vi "CH_LM DataString2StreamingCluster.vi"(3 "error in (no error)":errorcluster, 4 "Data Strings":string[](array[string]), 5 "Meter Index":i32) -> (0 "error out":errorcluster, 1 "Data Array":T1[](array[typedef]) {"Flags" format="%.0b"; "Unit ID" format="%.0b"; "Quad Distance"."Y" format="%#.1f"; "Quad Distance"."X" format="%#.1f"; "Value" format="%#.7e"}, 2 "Meter Index out":i32)   [LabVIEW 2017, in "CH_LM.lvlib"]
doc: "This VI converts the received data record strings to an array of Streaming Data Cluster."
uses:
  CH_LM.lvlib
  CH_LM/CH_LM Streaming Data.ctl
  CH_LM/CH_LM Data Token.ctl
panel:
  in  "Steaming Data Cluster":T1 {"Flags" format="%.0b"; "Unit ID" format="%.0b"; "Quad Distance"."Y" format="%#.1f"; "Quad Distance"."X" format="%#.1f"; "Value" format="%#.7e"}
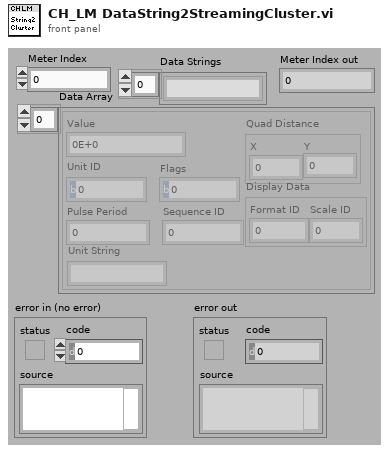
[diagram p1: front panel]
types:
  T1 = typedef "CH_LM.lvlib/CH_LM Streaming Data.ctl" = cluster{"Value":sgl, "Quad Distance":cluster{"X":sgl, "Y":sgl}, "Display Data":cluster{"Format ID":u8, "Scale ID":u8}, "Unit ID":u8, "Flags":u32, "Pulse Period":u32, "Sequence ID":u32, "Unit String":string}
  T2 = typedef "CH_LM.lvlib/CH_LM Data Token.ctl" = enum16{"Raw data", "Quad distance", "Formated data", "Unit", "Pulse period", "Flags", "Sequence ID"}
  T3 = typedef "CH_LM.lvlib/CH_LM Meter Info.ctl" = cluster{"Meter Index":i32, "Serial Number":string, "Queue Cluster":T4, "Data Header":bool, "Data Tokens":T2[]}
  T4 = typedef "CH_LM.lvlib/CH_LM Queue Cluster.ctl" = cluster{"Streaming Queue":refnum<queue>, "Asynch Notifier":refnum<notifier>}
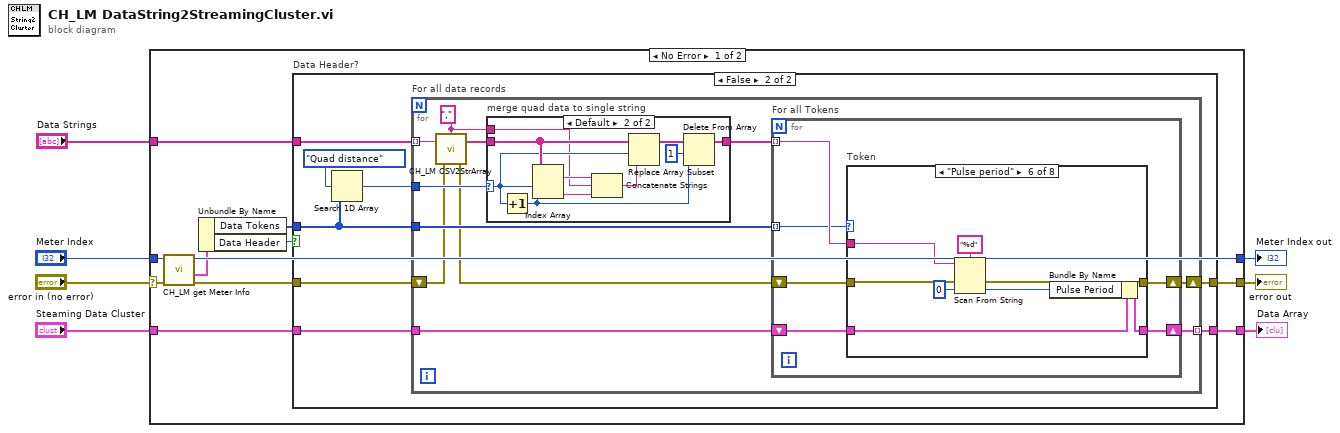
[diagram p0: block diagram]
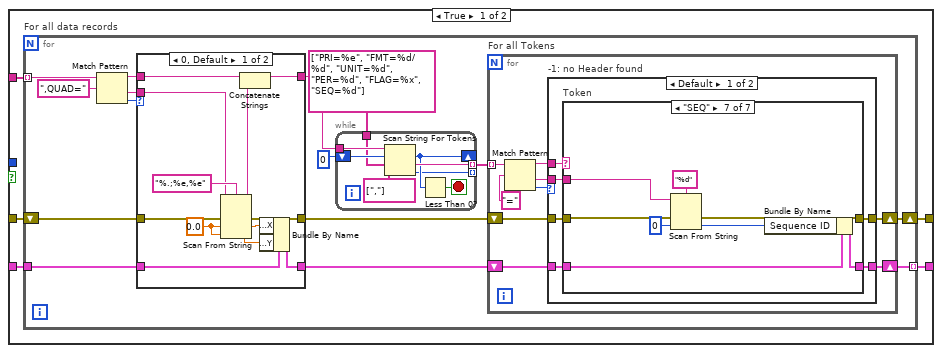
[diagram p2: hidden frame]
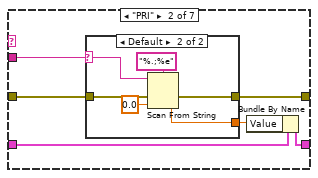
[diagram p5: hidden frame]
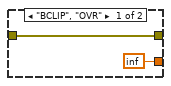
[diagram p6: hidden frame]
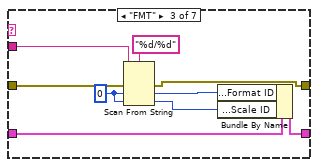
[diagram p7: hidden frame]
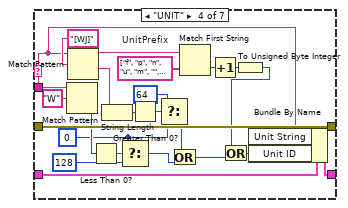
[diagram p8: hidden frame]
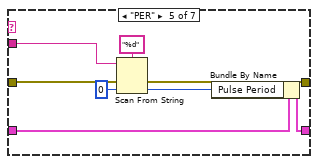
[diagram p9: hidden frame]
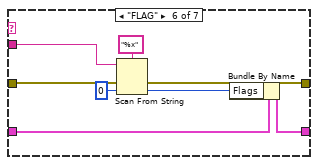
[diagram p10: hidden frame]
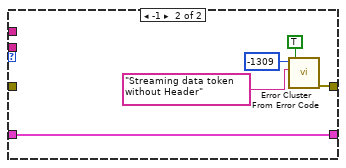
[diagram p11: hidden frame]
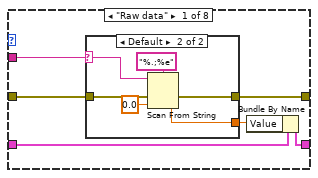
[diagram p13: hidden frame]
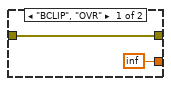
[diagram p14: hidden frame]
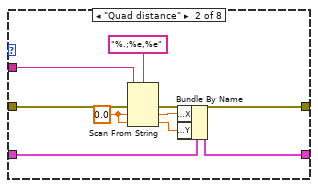
[diagram p15: hidden frame]
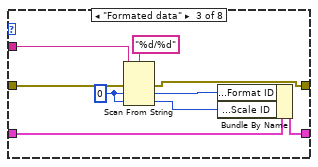
[diagram p16: hidden frame]
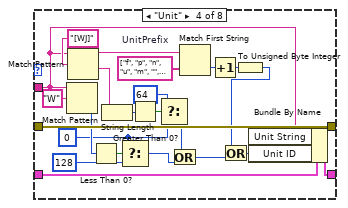
[diagram p17: hidden frame]
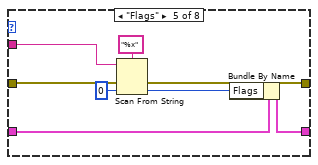
[diagram p18: hidden frame]
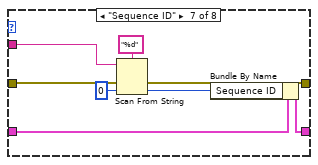
[diagram p19: hidden frame]
diagram:
  n1 = case shown="No Error" "error in (no error)" {
    selector: "error in (no error)" -> [w14 w272]
    tunnel: [w18 w272] -> w5
    tunnel: "Steaming Data Cluster" -> [w17 _]
    tunnel: [w16 _] -> w3
    tunnel: "Data Strings" -> [w15 _]
    tunnel: "Meter Index" -> [w12 w271]
    tunnel: [w11 w271] -> w1
    frame No Error {
      n2 = call "CH_LM get Meter Info.vi"("error in (no error)"=w14, "Meter Index"=w12) -> ("error out"=w13:errorcluster, "Meter Info"=w10:T3, "Meter Index out"=w11:i32)  [unwired: 7 out]
      n3 = Unbundle By Name(w10) -> ("Data Tokens"=w8:T2[], "Data Header"=w9:bool)
      n4 = case "Data Header?" shown="False" w9 {
        tunnel: [w23 w161] -> w18
        tunnel: w17 -> [w22 w160]
        tunnel: [w21 w159] -> w16
        tunnel: w15 -> [w20 w158]
        tunnel: w13 -> [w19 w157]
        tunnel: w8 -> [_ w156]
        frame True {
          n5 = for "For all data records" {
            tunnel: w22 -> [w27]
            tunnel: [w37] -> w21 mode=indexing
            tunnel: w20 -> [w33] mode=indexing
            shift-right: [w38] -> w23
            shift-left: w19 -> [w29]
            n6 = Match Pattern(string=w33, regular expression=",QUAD=") -> (before substring=w34:string, after substring=w30:string, offset past match=w25:i32)  [unwired: 2 out]
            n7 = case shown="0, Default" w25 {
              tunnel: w34 -> [w50 w53]
              tunnel: [w49 w53] -> w32
              tunnel: w30 -> [w44 _]
              tunnel: w29 -> [w43 w52]
              tunnel: [w42 w52] -> w28
              tunnel: w27 -> [w41 w51]
              tunnel: [w40 w51] -> w26
              frame 0, Default {
                w46 = sgl 0.0 ("default value 1")
                n8 = Scan From String(format string="%.;%e,%e", input string=w44, error in=w43, default 1=w46, default 2=w46) -> (remaining string=w39:string, error out=w42:errorcluster, output 1=w45:sgl, output 2=w47:sgl)  [unwired: 1 in, 1 out]
                n9 = Concatenate Strings(w50, w39) -> (w49:string)
                n10 = Bundle By Name(cluster=w41, "Quad Distance.X"=w45, "Quad Distance.Y"=w47) -> (w40:T1)
              }
              frame -1 {
              }
            }
            n11 = while {
              tunnel: w32 -> [w61]
              tunnel: [w60] -> w24 mode=indexing
              shift-right: [w57] -> _
              shift-left: 0 ("offset past token") -> [w59]
              tunnel: [w56] -> _ mode=indexing
              tunnel: string[] ["PRI=%e", "FMT=%d/%d", "UNIT=%d", "PER=%d", "FLAG=%x", "SEQ=%d"] ("operators (none)") -> [w54]
              stop <- w58 stop-if-true
              n12 = Scan String For Tokens(6:string[] [","] ("delimiters (\\s,\\t,\\r,\\n)"), 7:w54, 8:w59, 9:w61) -> (0:w56:i32, 1:w60:string, 2:w57:i32)  [unwired: 3 out]
              n13 = Less Than 0?(x=w57) -> (x < 0?=w58:bool)
            }
            n14 = for "For all Tokens" {
              tunnel: w24 -> [w69] mode=indexing
              shift-right: [w64] -> w37
              shift-left: w26 -> [w65]
              shift-right: [w62] -> w38
              shift-left: w28 -> [w63]
              n15 = Match Pattern(string=w69, regular expression="=") -> (before substring=w68:string, after substring=w66:string, offset past match=w67:i32)  [unwired: 2 out]
              n16 = case "-1: no Header found" shown="Default" w67 {
                tunnel: w68 -> [w76 _]
                tunnel: w66 -> [w75 _]
                tunnel: w65 -> [w74 w153]
                tunnel: [w73 w153] -> w64
                tunnel: w63 -> [w72 _]
                tunnel: [w71 w152] -> w62
                frame Default {
                  n17 = case "Token" shown="\"SEQ\"" w76 {
                    tunnel: w75 -> [_ w79 w101 w107 w130 w138 w146]
                    tunnel: w74 -> [w78 w84 w100 w124 w132 w140 w148]
                    tunnel: [w78 w82 w98 w123 w131 w139 w147] -> w73
                    tunnel: w72 -> [w77 w81 w94 w122 w125 w133 w142]
                    tunnel: [w77 w80 w93 w122 w126 w134 w141] -> w71
                    frame Default {
                    }
                    frame "PRI" {
                      n18 = case shown="Default" w79 {
                        selector: w79 -> [_ w87]
                        tunnel: [sgl inf w92] -> w83
                        tunnel: w81 -> [w86 w89]
                        tunnel: [w86 w88] -> w80
                        frame "BCLIP", "OVR" {
                        }
                        frame Default {
                          n19 = Scan From String(format string="%.;%e", input string=w87, error in=w89, default 1=sgl 0.0 ("default value 1")) -> (error out=w88:errorcluster, output 1=w92:sgl)  [unwired: 1 in, 2 out]
                        }
                      }
                      n20 = Bundle By Name(cluster=w84, "Value"=w83) -> (w82:T1)
                    }
                    frame "FMT" {
                      w97 = u8 0 ("default value 1")
                      n21 = Scan From String(format string="%d/%d", input string=w101, error in=w94, default 1=w97, default 2=w97) -> (error out=w93:errorcluster, output 1=w99:u8, output 2=w96:u8)  [unwired: 1 in, 2 out]
                      n22 = Bundle By Name(cluster=w100, "Display Data.Format ID"=w99, "Display Data.Scale ID"=w96) -> (w98:T1)
                    }
                    frame "UNIT" {
                      w111 = string[] ["f", "p", "n", "u", "m", "", "k", "M", "G", "T", "P"]  # UnitPrefix
                      w114 = u8 0 ("default value 1")
                      n23 = Match Pattern(string=w107, regular expression="W") -> (offset past match=w120:i32)  [unwired: 4 out]
                      n24 = Match Pattern(string=w107, regular expression="[WJ]") -> (before substring=w108:string, after substring=w109:string)  [unwired: 3 out]
                      n25 = Less Than 0?(x=w120) -> (x < 0?=w119:bool)
                      n26 = String Length(string=w109) -> (length=w117:i32)
                      n27 = Select(t=w114, s=w119, f=u8 128 ("default value 1")) -> (s? t:f=w112:u8)
                      n28 = Greater Than 0?(x=w117) -> (x > 0?=w116:bool)
                      n29 = Select(t=u8 64 ("default value 1"), s=w116, f=w114) -> (s? t:f=w113:u8)
                      n30 = Or(x=w113, y=w112) -> (x .or. y?=w105:u8)
                      n31 = Match First String(2:w111, 3:w108) -> (0:w106:i32)  [unwired: 1 out]
                      n32 = Increment(x=w106) -> (x+1=w102:i32)
                      n33 = To Unsigned Byte Integer(number=w102) -> (unsigned 8bit integer=w103:u8)
                      n34 = Or(x=w103, y=w105) -> (x .or. y?=w104:u8)
                      n35 = Bundle By Name(cluster=w124, "Unit String"=w107, "Unit ID"=w104) -> (w123:T1)
                    }
                    frame "PER" {
                      n36 = Scan From String(format string="%d", input string=w130, error in=w125, default 1=u32 0 ("default value 1")) -> (error out=w126:errorcluster, output 1=w129:u32)  [unwired: 1 in, 2 out]
                      n37 = Bundle By Name(cluster=w132, "Pulse Period"=w129) -> (w131:T1)
                    }
                    frame "FLAG" {
                      n38 = Scan From String(format string="%x", input string=w138, error in=w133, default 1=u8 0 ("default value 1")) -> (error out=w134:errorcluster, output 1=w137:u8)  [unwired: 1 in, 2 out]
                      n39 = Bundle By Name(cluster=w140, "Flags"=w137) -> (w139:T1)
                    }
                    frame "SEQ" {
                      n40 = Scan From String(format string="%d", input string=w146, error in=w142, default 1=u32 0 ("default value 1")) -> (error out=w141:errorcluster, output 1=w145:u32)  [unwired: 1 in, 2 out]
                      n41 = Bundle By Name(cluster=w148, "Sequence ID"=w145) -> (w147:T1)
                    }
                  }
                }
                frame -1 {
                  n42 = call <vilib>:"Error Cluster From Error Code.vi"("show call chain? (False)"=TRUE, "error message (\"\")"="Streaming data token without Header" ("error message (\"\")"), "error code (0)"=-1309) -> ("error out"=w152:errorcluster)  [unwired: 1 in, 5 out]
                }
              }
            }
          }
        }
        frame False {
          n43 = Search 1D Array(1D array=w156, element=CH_LM_Data_Token."Quad distance" ("Data Token")) -> (index of element=w154:i32)  [unwired: 1 out]
          n44 = for "For all data records" {
            tunnel: w160 -> [w170]
            tunnel: [w171] -> w159 mode=indexing
            tunnel: w158 -> [w169] mode=indexing
            shift-right: [w172] -> w161
            shift-left: w157 -> [w164]
            tunnel: w156 -> [w168]
            tunnel: w154 -> [w165]
            w162 = "," ("Separator (,)")
            n45 = call "CH_LM CSV2StrArray.vi"("error in (no error)"=w164, "CSL"=w169, "Separator (,)"=w162) -> ("error out"=w163:errorcluster, "Strings"=w167:string[])
            n46 = case "merge quad data to single string" shown="Default" w165 {
              selector: w165 -> [_ w175]
              tunnel: w167 -> [w173 w181]
              tunnel: [w173 w178] -> w166
              tunnel: w162 -> [_ w174]
              frame -1 {
              }
              frame Default {
                n47 = Increment(x=w175) -> (x+1=w177:i32)
                n48 = Index Array(array=w181, index #1=w175, index #2=w177) -> (element #1=w182:string, element #2=w183:string)
                n49 = Concatenate Strings(w182, w174, w183) -> (w180:string)
                n50 = Replace Array Subset(array=w181, new element=w180, index=w175) -> (w179:string[])
                n51 = Delete From Array(array=w179, length=1, index=w177) -> (array with subset deleted=w178:string[])  [unwired: 1 out]
              }
            }
            n52 = for "For all Tokens" {
              shift-right: [w188] -> w171
              shift-left: w170 -> [w189]
              shift-right: [w186] -> w172
              shift-left: w163 -> [w187]
              tunnel: w166 -> [w185] mode=indexing
              tunnel: w168 -> [w184] mode=indexing
              n53 = case "Token" shown="\"Pulse period\"" w184 {
                tunnel: w185 -> [w190 w204 w221 w227 w250 w258 w266 _]
                tunnel: w189 -> [w195 w206 w220 w244 w252 w260 w268 w270]
                tunnel: [w193 w207 w218 w243 w251 w259 w267 w270] -> w188
                tunnel: w187 -> [w192 w209 w214 w242 w245 w253 w262 w269]
                tunnel: [w191 w208 w213 w242 w246 w254 w261 w269] -> w186
                frame "Raw data" {
                  n54 = case shown="Default" w190 {
                    selector: w190 -> [_ w198]
                    tunnel: [sgl inf w203] -> w194
                    tunnel: w192 -> [w197 w200]
                    tunnel: [w197 w199] -> w191
                    frame "BCLIP", "OVR" {
                    }
                    frame Default {
                      n55 = Scan From String(format string="%.;%e", input string=w198, error in=w200, default 1=sgl 0.0 ("default value 1")) -> (error out=w199:errorcluster, output 1=w203:sgl)  [unwired: 1 in, 2 out]
                    }
                  }
                  n56 = Bundle By Name(cluster=w195, "Value"=w194) -> (w193:T1)
                }
                frame "Quad distance" {
                  w211 = sgl 0.0 ("default value 1")
                  n57 = Scan From String(format string="%.;%e,%e", input string=w204, error in=w209, default 1=w211, default 2=w211) -> (error out=w208:errorcluster, output 1=w210:sgl, output 2=w205:sgl)  [unwired: 1 in, 2 out]
                  n58 = Bundle By Name(cluster=w206, "Quad Distance.X"=w210, "Quad Distance.Y"=w205) -> (w207:T1)
                }
                frame "Formated data" {
                  w217 = u8 0 ("default value 1")
                  n59 = Scan From String(format string="%d/%d", input string=w221, error in=w214, default 1=w217, default 2=w217) -> (error out=w213:errorcluster, output 1=w219:u8, output 2=w216:u8)  [unwired: 1 in, 2 out]
                  n60 = Bundle By Name(cluster=w220, "Display Data.Format ID"=w219, "Display Data.Scale ID"=w216) -> (w218:T1)
                }
                frame "Unit" {
                  w231 = string[] ["f", "p", "n", "u", "m", "", "k", "M", "G", "T", "P"]  # UnitPrefix
                  w234 = u8 0 ("default value 1")
                  n61 = Match Pattern(string=w227, regular expression="W") -> (offset past match=w240:i32)  [unwired: 4 out]
                  n62 = Match Pattern(string=w227, regular expression="[WJ]") -> (before substring=w228:string, after substring=w229:string)  [unwired: 3 out]
                  n63 = Less Than 0?(x=w240) -> (x < 0?=w239:bool)
                  n64 = String Length(string=w229) -> (length=w237:i32)
                  n65 = Select(t=w234, s=w239, f=u8 128 ("default value 1")) -> (s? t:f=w232:u8)
                  n66 = Greater Than 0?(x=w237) -> (x > 0?=w236:bool)
                  n67 = Select(t=u8 64 ("default value 1"), s=w236, f=w234) -> (s? t:f=w233:u8)
                  n68 = Or(x=w233, y=w232) -> (x .or. y?=w225:u8)
                  n69 = Match First String(2:w231, 3:w228) -> (0:w226:i32)  [unwired: 1 out]
                  n70 = Increment(x=w226) -> (x+1=w222:i32)
                  n71 = To Unsigned Byte Integer(number=w222) -> (unsigned 8bit integer=w223:u8)
                  n72 = Or(x=w223, y=w225) -> (x .or. y?=w224:u8)
                  n73 = Bundle By Name(cluster=w244, "Unit String"=w227, "Unit ID"=w224) -> (w243:T1)
                }
                frame "Flags" {
                  n74 = Scan From String(format string="%x", input string=w250, error in=w245, default 1=u8 0 ("default value 1")) -> (error out=w246:errorcluster, output 1=w249:u8)  [unwired: 1 in, 2 out]
                  n75 = Bundle By Name(cluster=w252, "Flags"=w249) -> (w251:T1)
                }
                frame "Pulse period" {
                  n76 = Scan From String(format string="%d", input string=w258, error in=w253, default 1=u32 0 ("default value 1")) -> (error out=w254:errorcluster, output 1=w257:u32)  [unwired: 1 in, 2 out]
                  n77 = Bundle By Name(cluster=w260, "Pulse Period"=w257) -> (w259:T1)
                }
                frame "Sequence ID" {
                  n78 = Scan From String(format string="%d", input string=w266, error in=w262, default 1=u32 0 ("default value 1")) -> (error out=w261:errorcluster, output 1=w265:u32)  [unwired: 1 in, 2 out]
                  n79 = Bundle By Name(cluster=w268, "Sequence ID"=w265) -> (w267:T1)
                }
                frame Default {
                }
              }
            }
          }
        }
      }
    }
    frame Error {
    }
  }
  "error out" <- w5
  "Data Array" <- w3
  "Meter Index out" <- w1
